vi "Close.vi"(8 "Error In":errorcluster, 11 "VISA Resource in":refnum<visa-resource-name>) -> (0 "Error Out":errorcluster)   [LabVIEW 2016, in "KIT QV.lvlib"]
doc: "Close connection to the instrument."
uses:
  KIT QV.lvlib
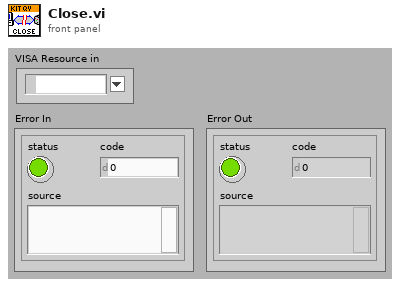
[diagram p1: front panel]
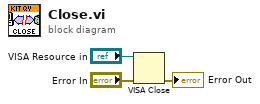
[diagram p0: block diagram]
diagram:
  n1 = VISA Close(VISA resource name="VISA Resource in", error in (no error)="Error In") -> (error out=→"Error Out":errorcluster)
